vi "Set Attributes.vi"(8 "error in (no error)":errorcluster, 10 "Attributes":T1={"Expires"=timestamp(0 s since 1904-01-01), "Secure"=FALSE, "HttpOnly"=TRUE, "Domain"="", "Path"="", "SameSite"=enum."Unset (Lax)", "Prefix"=enum."None", "Max-Age Expiry"=TRUE}, 11 "Cookie in":refnum<class "Cookie.lvclass">) -> (0 "error out":errorcluster, 3 "Cookie out":refnum<class "Cookie.lvclass">)   [LabVIEW 2020, in "HTTP Utils.lvlib" / "Cookie.lvclass"]
uses:
  Cookie.lvclass
  Cookie SameSite.ctl
  HTTP Utils.lvlib
  Cookie Prefix.ctl
  Cookie Attributes.ctl
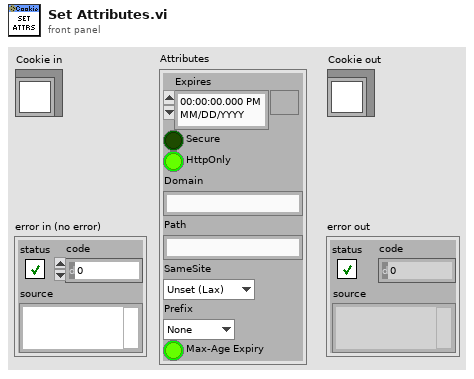
[diagram p1: front panel]
types:
  T1 = typedef "HTTP Utils.lvlib/Cookie Attributes.ctl" = cluster{"Expires":timestamp, "Secure":bool, "HttpOnly":bool, "Domain":string, "Path":string, "SameSite":T2, "Prefix":T3, "Max-Age Expiry":bool}
  T2 = typedef "HTTP Utils.lvlib/Cookie SameSite.ctl" = enum16{"Unset (Lax)", "Lax", "Strict", "None"}
  T3 = typedef "HTTP Utils.lvlib/Cookie Prefix.ctl" = enum16{"None", "Host", "Secure"}
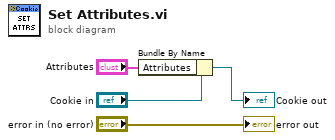
[diagram p0: block diagram]
diagram:
  n1 = Bundle By Name(cluster="Cookie in", "Attributes"="Attributes") -> (→"Cookie out":refnum<class "Cookie.lvclass">)
  "error out" <- "error in (no error)"
